vi "Acad NET ready.vi"(10 "error in (no error)":errorcluster, 11 "AutoCad app in":refnum<k24>) -> (2 "error out":errorcluster, 3 "AutoCAD app out":refnum<k24>, 5 "seconds since 1Jan1904":timestamp)   [LabVIEW 2011, in "Design Server.lvlib"]
uses:
  Design Server.lvlib
  C:/Program Files/Autodesk/AutoCAD 2013/Autodesk.AutoCAD.Interop.dll
  Program Files/Autodesk/AutoCAD 2013/Autodesk.AutoCAD.Interop.dll
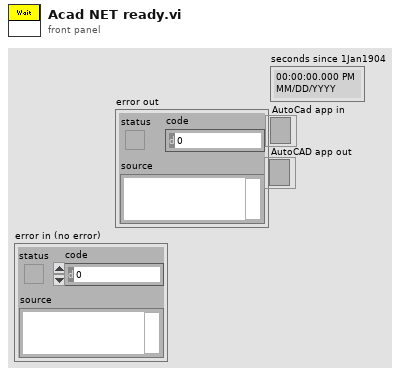
[diagram p1: front panel]
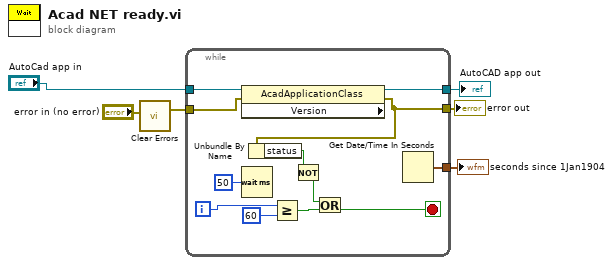
[diagram p0: block diagram]
diagram:
  n1 = call <vilib>:"Clear Errors.vi"("error in (no error)"="error in (no error)") -> ("error out"=w3:errorcluster)  [unwired: 6 in]
  n2 = while {
    tunnel: "AutoCad app in" -> [w18]
    tunnel: [w17] -> w1
    tunnel: [w15] -> w6
    tunnel: w3 -> [w16]
    tunnel: [w8] -> w4
    i -> [w11]
    stop <- w14 stop-if-true
    n3 = property class="AcadApplicationClass" props=["Version"](reference=w18, error in=w16) -> (reference out=w17:refnum<k24>, error out=w15:errorcluster)  [unwired: 1 out]
    n4 = Wait (ms)(milliseconds to wait=u32 50) -> ()  [unwired: 1 out]
    n5 = Unbundle By Name(w15) -> ("status"=w13:bool)
    n6 = Greater Or Equal?(x=w11, y=60) -> (x >= y?=w10:bool)
    n7 = Not(x=w13) -> (.not. x?=w7:bool)
    n8 = Or(x=w7, y=w10) -> (x .or. y?=w14:bool)
    n9 = Get Date/Time In Seconds() -> (seconds since 1Jan1904=w8:timestamp)
  }
  "error out" <- w6
  "seconds since 1Jan1904" <- w4
  "AutoCAD app out" <- w1
